vi "图片录入.vi"(9 "身份证":string, 11 "Image 2":T1(plugin-control)) -> (2 "photoid":string)   [LabVIEW 2013]
panel:
  out "Image":T1(plugin-control)
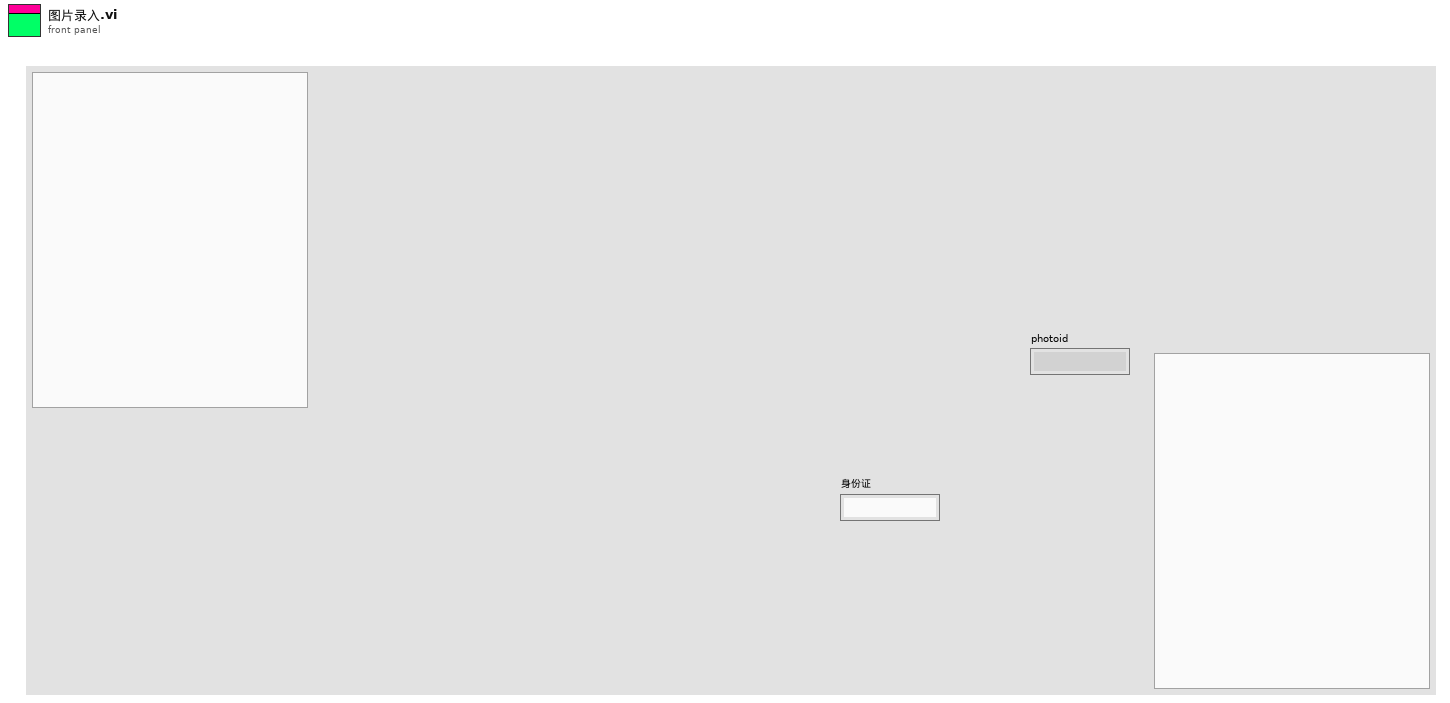
[diagram p1: front panel]
types:
  T1 = typedef "IMAQ Image.ctl" = refnum<image>
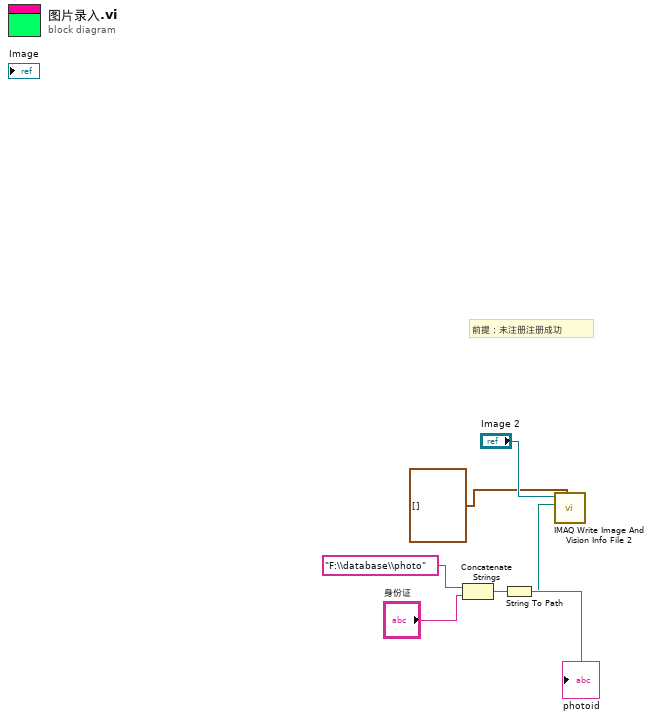
[diagram p0: block diagram]
diagram:
  # "前提：未注册注册成功"
  n1 = Concatenate Strings("F:\\database\\photo" ("身份证"), "身份证") -> (w2:string)
  "photoid" <- w2
  n2 = String To Path(string=w2) -> (path=w1:path)
  n3 = call "IMAQ Write Image And Vision Info File 2"("Color Palette"=cluster{"Red":u8, "Green":u8, "Blue":u8}[] [], "File Path"=w1, "Image"="Image 2") -> ()  [unwired: 7 in, 2 out]
